vi "liberror.vi"(10 "tvio errors":T1, 11 "error in (no error)":errorcluster) -> (3 "error out":errorcluster)   [LabVIEW 2015]
uses:
  error.ctl
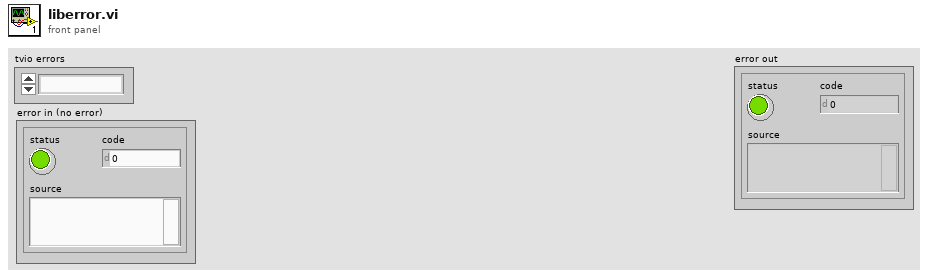
[diagram p1: front panel]
types:
  T1 = typedef "error.ctl" = enum16{"", "ERR_INVALID_DESCRIPTOR", "ERR_INVALID_INPUT", "ERR_INVALID_OUTPUT", "ERR_INVALID_RESULT_ID", "ERR_INVALID_REQUEST_ID", "ERR_NO_RESULT_AVAILABLE", "ERR_RESULT_NOT_ARRIVED"}
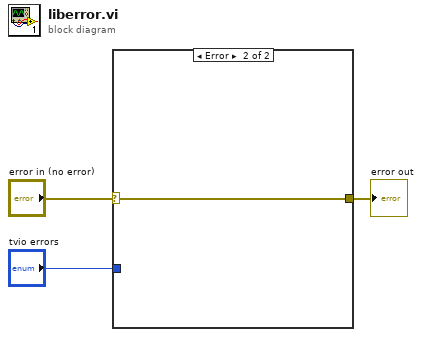
[diagram p0: block diagram]
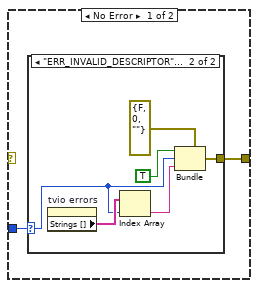
[diagram p2: hidden frame]
diagram:
  n1 = case shown="Error" "error in (no error)" {
    selector: "error in (no error)" -> [_ w12]
    tunnel: "tvio errors" -> [w5 _]
    tunnel: [w4 w12] -> w1
    frame No Error {
      n2 = case shown="\"ERR_INVALID_DESCRIPTOR\", Default" w5 {
        selector: w5 -> [_ w8]
        tunnel: [_ w6] -> w4
        frame "" {
        }
        frame "ERR_INVALID_DESCRIPTOR", Default {
          n3 = property on="tvio errors" class="Enum (strict)"() -> ("Strings []"=w11:string[])  [unwired: 2 in, 2 out]
          n4 = Index Array(array=w11, index=w8) -> (element=w7:string)
          n5 = Bundle(cluster=errorcluster {"status"=FALSE, "code"=0, "source"=""} ("error out"), "status"=TRUE, "code"=w8, "source"=w7) -> (w6:errorcluster)
        }
      }
    }
    frame Error {
    }
  }
  "error out" <- w1
